vi "ConditionsGlobal.vi"() -> ()   [LabVIEW 2014]
panel:
  out "SMConnected":bool
  out "NIConnected":bool
  out "ArduinoConnected":bool
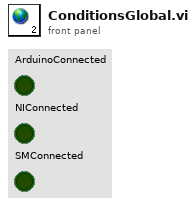
[diagram p1: front panel]
diagram:
